vi "Add Commit Menu.vi"(8 "error in":errorcluster, 9 "Commit ID":i32, 10 "LabVIEW Files?":bool[](array[boolean]), 11 "Menu Ref":refnum<k9>) -> (0 "error out":errorcluster)   [LabVIEW 2020, in "Peer Review.lvclass"]
uses:
  Peer Review.lvclass
  Peer Review.lvclass/Peer Review.ctl
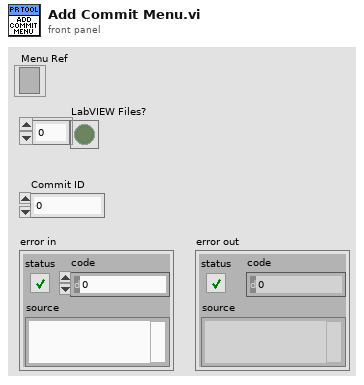
[diagram p1: front panel]
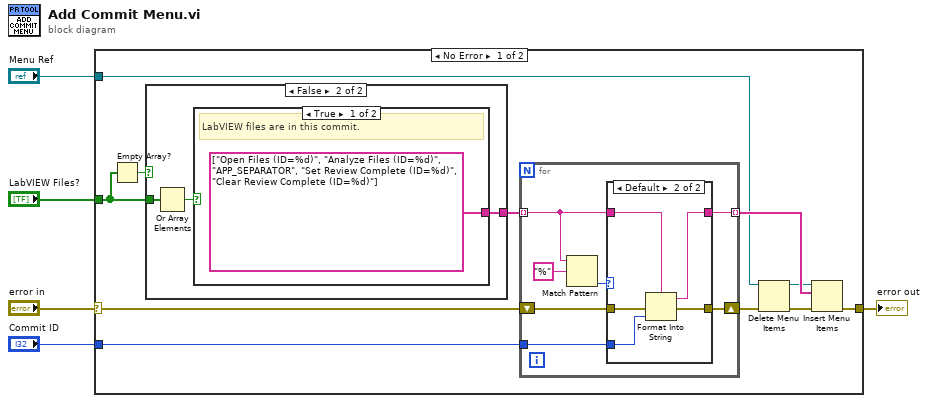
[diagram p0: block diagram]
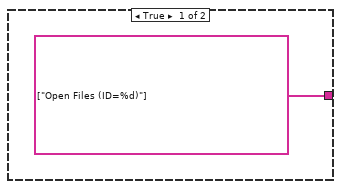
[diagram p2: hidden frame]
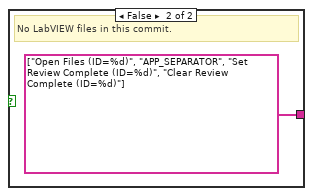
[diagram p3: hidden frame]
diagram:
  n1 = case shown="No Error" "error in" {
    selector: "error in" -> [w11 w37]
    tunnel: "LabVIEW Files?" -> [w7 _]
    tunnel: [w10 w37] -> w4
    tunnel: "Menu Ref" -> [w9 _]
    tunnel: "Commit ID" -> [w8 _]
    frame No Error {
      n2 = Empty Array?(array=w7) -> (empty?=w6:bool)
      n3 = case shown="False" w6 {
        tunnel: [string[] ["Open Files (ID=%d)"] ("format string") w20] -> w15
        tunnel: w7 -> [_ w18]
        frame True {
        }
        frame False {
          n4 = Or Array Elements(Boolean array=w18) -> (logical OR=w19:bool)
          n5 = case shown="True" w19 {
            tunnel: [string[] ["Open Files (ID=%d)", "Analyze Files (ID=%d)", "APP_SEPARATOR", "Set Review Complete (ID=%d)", "Clear Review Complete (ID=%d)"] ("format string") string[] ["Open Files (ID=%d)", "APP_SEPARATOR", "Set Review Complete (ID=%d)", "Clear Review Complete (ID=%d)"] ("format string")] -> w20
            frame True {
              # "LabVIEW files are in this commit."
            }
            frame False {
              # "No LabVIEW files in this commit."
            }
          }
        }
      }
      n6 = for {
        tunnel: w8 -> [w29]
        tunnel: w15 -> [w24] mode=indexing
        shift-right: [w28] -> w13
        shift-left: w11 -> [w27]
        tunnel: [w26] -> w16 mode=indexing
        n7 = Match Pattern(string=w24, regular expression="%") -> (offset past match=w23:i32)  [unwired: 1 in, 3 out]
        n8 = case shown="Default" w23 {
          tunnel: w29 -> [_ w36]
          tunnel: [w30 w35] -> w28
          tunnel: w27 -> [w30 w34]
          tunnel: [w31 w33] -> w26
          tunnel: w24 -> [w31 w32]
          frame -1 {
            # "For separator\nline"
          }
          frame Default {
            n9 = Format Into String(format string=w32, error in=w34, w36) -> (resulting string=w33:string, error out=w35:errorcluster)  [unwired: 1 in]
          }
        }
      }
      n10 = Delete Menu Items(6:w13, 9:w9) -> (0:w14:errorcluster, 3:w12:refnum<k9>)  [unwired: 2 in]
      n11 = Insert Menu Items(6:w14, 8:w16, 9:w12) -> (0:w10:errorcluster)  [unwired: 3 in, 2 out]
    }
    frame Error {
    }
  }
  "error out" <- w4
